vi "tb_logarith_dsp48e.vi"() -> ()   [LabVIEW 2011]
uses:
  <vilib>/Analysis/NI_AALBase.lvlib
  <vilib>/Analysis/1siggen.llb/Ramp Pattern by Samples.vi
panel:
  out "Max Error":dbl=0.017273251214031227
  in  "Number of Test Points":i32=16384
  out "FLP":dbl[](array[numeric])
  out "FXP":dbl[](array[numeric])
  out "Error Signal":dbl[](graph)
  out "Exponent (-N)":i8=-1
  out "Mantissa (M)":fxp<+,32,0>=0.5 format="%.0b"
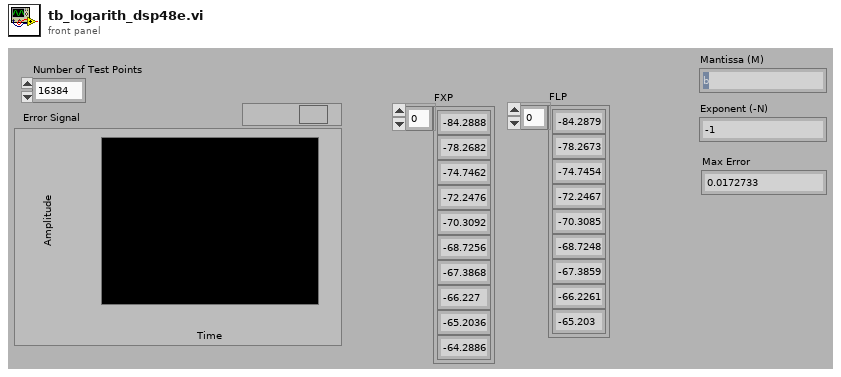
[diagram p1: front panel]
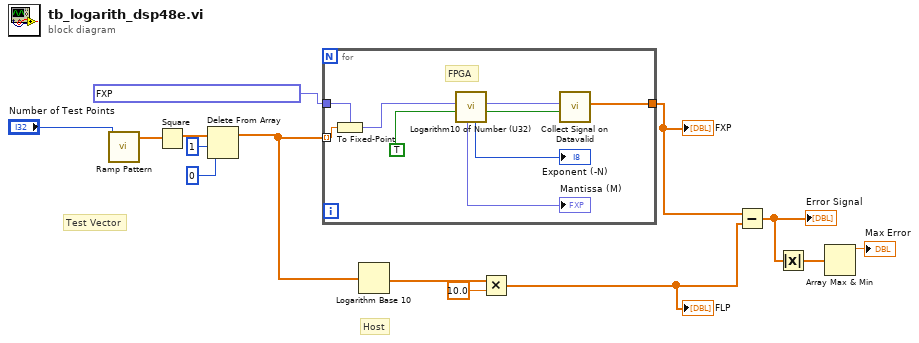
[diagram p0: block diagram]
diagram:
  # "Host"
  # "Test Vector"
  n1 = call-poly <vilib>:"Ramp Pattern.vi"("samples"="Number of Test Points") -> ("Ramp Pattern"=w10:dbl[])  [unwired: 9 in, 1 out]
  n2 = Square(x=w10) -> (x^2=w7:dbl[])
  n3 = Delete From Array(array=w7, length=1, index=0) -> (array with subset deleted=w6:dbl[])  [unwired: 1 out]
  n4 = for {
    tunnel: fxp<+,32,1> 0.0 ("Input Number (1.32)") -> [w18]
    tunnel: [w20] -> w9
    tunnel: w6 -> [w16] mode=indexing
    # "FPGA"
    n5 = To Fixed-Point(fixed-point type=w18, number=w16) -> (fixed-point=w17:fxp<+,32,1>)
    n6 = call <userlib>:"Logarithm10 of Number (U32).vi"("Input Valid"=TRUE, "Input Number (0.32)"=w17) -> ("Output Valid"=w21:bool, "Logarithm"=w22:fxp<+/-,34,12>, "Exponent (-N)"=→"Exponent (-N)":i8, "Mantissa (M)"=→"Mantissa (M)":fxp<+,32,0>)  [unwired: 6 in]
    n7 = call <userlib>:"Collect Signal on Datavalid.vi"("Data Valid"=w21, "Input"=w22) -> ("Output"=w20:dbl[])  [unwired: 9 in]
  }
  "FXP" <- w9
  n8 = Logarithm Base 10(1:w6) -> (0:w13:dbl[])
  n9 = Multiply(x=w13, y=10.0) -> (x*y=w8:dbl[])
  "FLP" <- w8
  n10 = Subtract(x=w9, y=w8) -> (x-y=w3:dbl[])
  "Error Signal" <- w3
  n11 = Absolute Value(x=w3) -> (abs(x)=w2:dbl[])
  n12 = Array Max & Min(array=w2) -> (max value=→"Max Error":dbl)  [unwired: 3 out]
